vi "RoutineData.vi"() -> ()   [LabVIEW 2017]
panel:
  in  "DrivePath":cluster{"Path":string}
  in  "DriveForDistance":cluster{"Distance":dbl, "Speed":dbl}
  in  "Wait":cluster{"Time":u32}
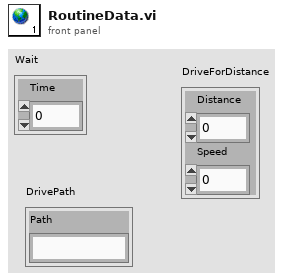
[diagram p1: front panel]
diagram:
